vi "Calculate execution time for scans.vi"(8 "error in (no error)":errorcluster, 11 "Command string IN":string) -> (0 "error out":errorcluster, 3 "Execution time":dbl)   [LabVIEW 2012]
doc: "SciScan 1.2 160622"
uses:
  INI/settingsIO/Settings IO_Commands.ctl
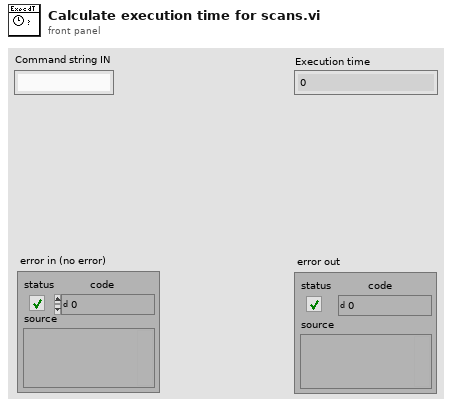
[diagram p1: front panel]
types:
  T1 = typedef "Setting File Types.ctl" = enum16{"2D.Frame.Scan.Settings", "2D.Line.Scan.Settings", "Z.Stack.Settings", "HW Settings", "Configuration Settings", "Unknown Settings", "Fast.Z.Settings"}
  T2 = typedef "Settings IO_Commands.ctl" = enum16{"Write HW Settings", "Write Config Settings", "Read HW Settings", "Read Config Settings", "Write Line-Scan Settings", "Write Frame-Scan Settings", "Write Z-Stack Settings", "Read Line-Scan Settings", "Read Frame-Scan Settings", "Read Z-Stack Settings", "Read Fast-Z Settings", "Write Fast-Z Settings"}
  T3 = typedef "GFG Variable for IO.ctl" = cluster{"Variable Name":string, "Value (Variant)":variant, "data type":string}
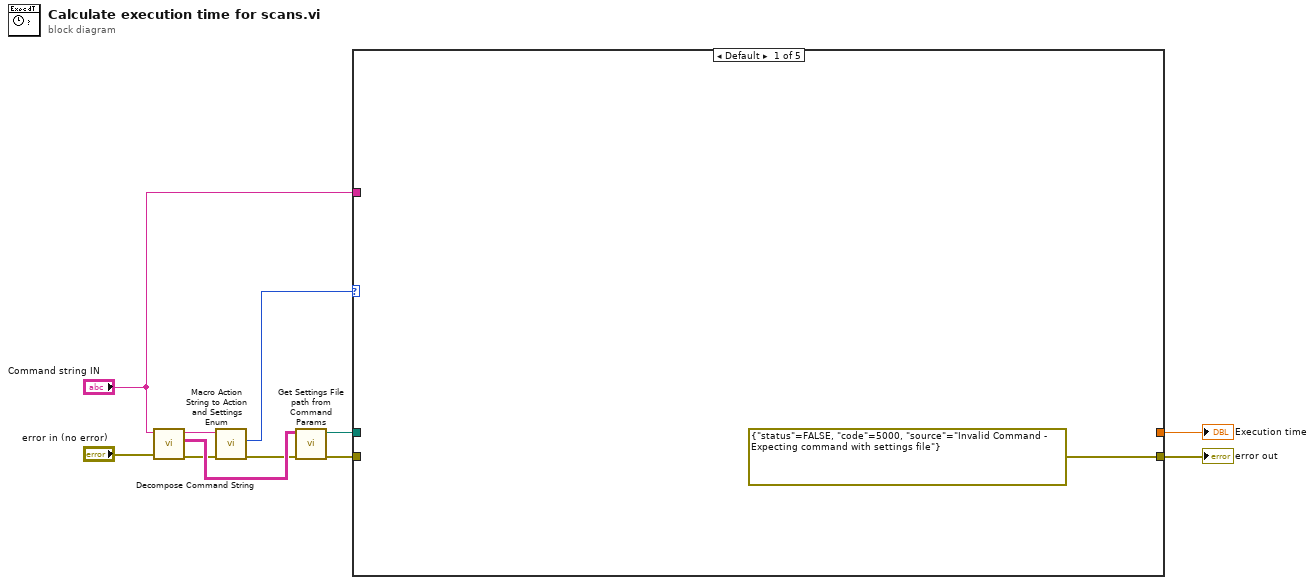
[diagram p0: block diagram]
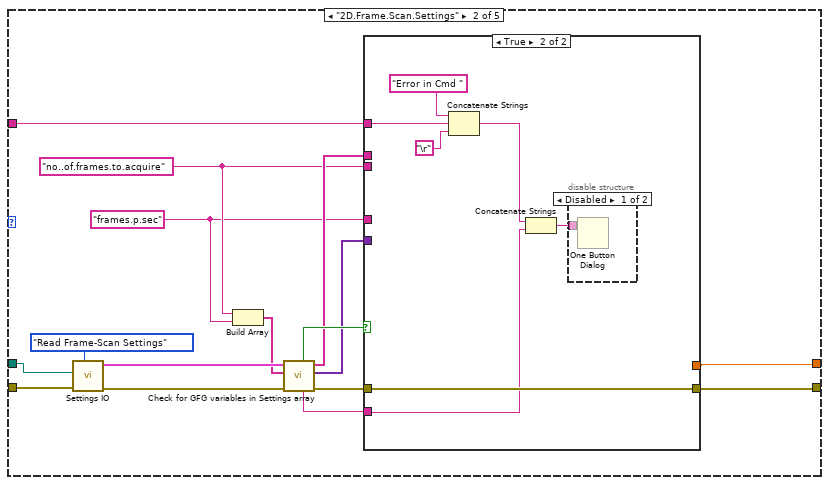
[diagram p2: hidden frame]
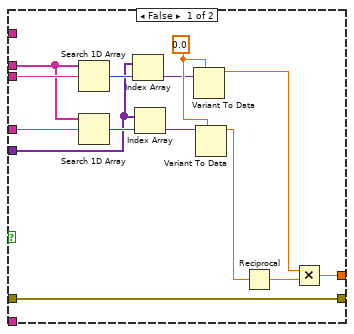
[diagram p3: hidden frame]
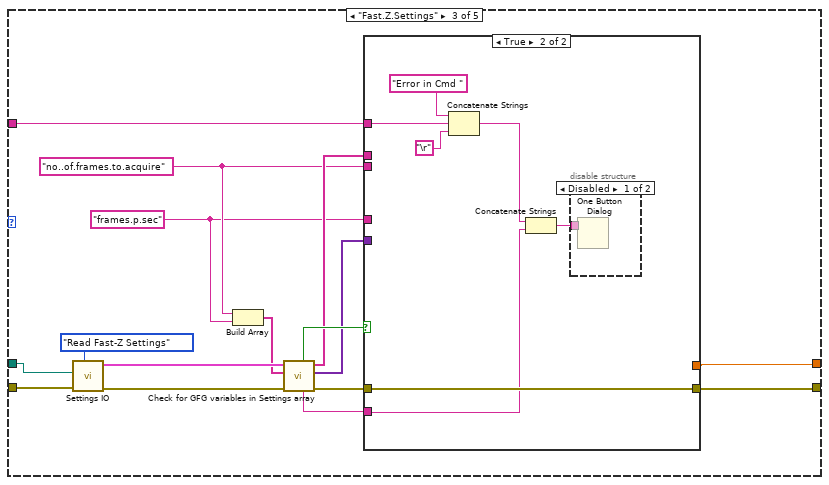
[diagram p5: hidden frame]
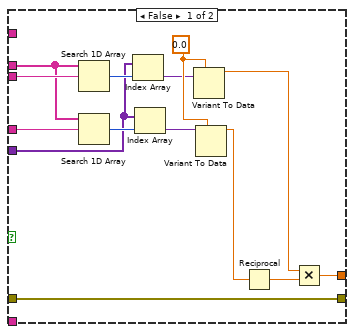
[diagram p6: hidden frame]
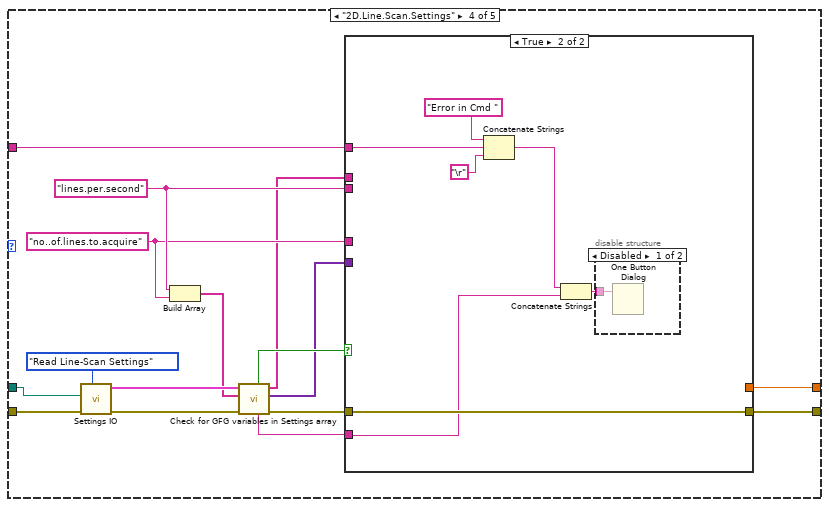
[diagram p8: hidden frame]
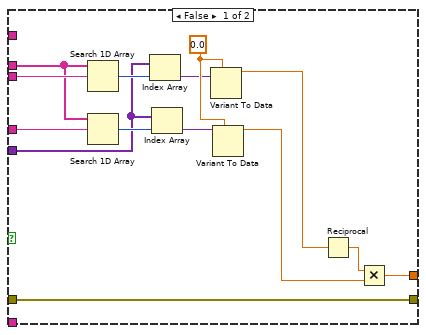
[diagram p9: hidden frame]
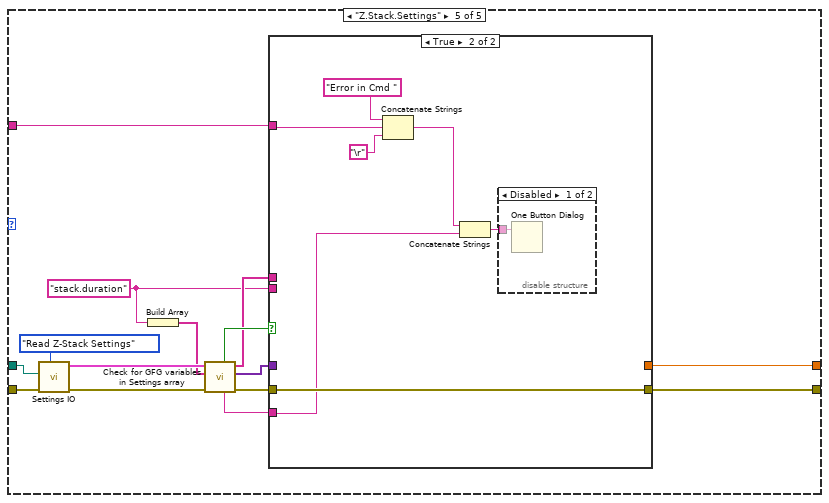
[diagram p11: hidden frame]
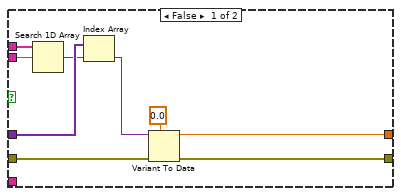
[diagram p12: hidden frame]
diagram:
  n1 = call "Decompose Command String.vi"("Error In"="error in (no error)", "Command IN"="Command string IN") -> ("Error Out"=w10:errorcluster, "Parameter Table"=w11:string[][], "Action"=w9:string)  [unwired: 6 in, 1 out]
  n2 = call "Macro Action String to Action and Settings Enum.vi"("error in (no error)"=w10, "Action String IN"=w9) -> ("error out"=w8:errorcluster, "Setting File Type OUT"=w7:T1)  [unwired: 6 in, 2 out]
  n3 = call "Get Settings File path from Command Params.vi"("error in (no error)"=w8, "Params Array IN"=w11) -> ("error out"=w5:errorcluster, "Settings Path OUT"=w6:path)  [unwired: 8 in]
  n4 = case shown="Default" w7 {
    tunnel: w6 -> [_ w23 w61 w102 w139]
    tunnel: w5 -> [_ w24 w62 w103 w140]
    tunnel: [errorcluster {"status"=FALSE, "code"=5000, "source"="Invalid Command - Expecting command with settings file"} ("error constant") w22 w60 w95 w133] -> w2
    tunnel: [_ w14 w52 w94 w132] -> w4
    tunnel: "Command string IN" -> [_ w13 w51 w89 w127]
    frame Default {
    }
    frame "2D.Frame.Scan.Settings" {
      w17 = "no..of.frames.to.acquire" ("Command string IN 2")
      w16 = "frames.p.sec" ("Command string IN 2")
      n5 = call "Settings IO.vi"("SettingsFileIO_Commands"=Settings_IO_Commands."Read Frame-Scan Settings", "Error In"=w24, "File Path (for scan specific settings)"=w23) -> ("Error Out"=w26:errorcluster, "Settings Array OUT"=w27:T3[])  [unwired: 6 in, 1 out]
      n6 = Build Array(w17, w16) -> (w25:string[])
      n7 = call "Check for GFG variables in Settings array.vi"("error in (no error)"=w26, "GFG variables to search"=w25, "Settings ArrayIN"=w27) -> ("error out"=w21:errorcluster, "GFG variant values (those found)"=w15:variant[], "GFG variables found"=w18:string[], "Error Message (list of variables not found)"=w19:string, "Any Not Found?"=w20:bool)  [unwired: 3 in, 1 out]
      n8 = case shown="True" w20 {
        tunnel: w19 -> [_ w44]
        tunnel: w21 -> [w42 w49]
        tunnel: [w42 w49] -> w22
        tunnel: [w41 _] -> w14
        tunnel: w17 -> [w35 _]
        tunnel: w16 -> [w34 _]
        tunnel: w18 -> [w33 _]
        tunnel: w15 -> [w32 _]
        tunnel: w13 -> [_ w47]
        frame False {
          w40 = 0.0 ("x*y")
          n9 = Search 1D Array(1D array=w33, element=w35) -> (index of element=w37:i32)  [unwired: 1 in]
          n10 = Search 1D Array(1D array=w33, element=w34) -> (index of element=w36:i32)  [unwired: 1 in]
          n11 = Index Array(array=w32, index=w37) -> (element=w39:variant)
          n12 = Index Array(array=w32, index=w36) -> (element=w38:variant)
          n13 = Variant To Data(type=w40, Variant=w39) -> (data=w31:dbl)  [unwired: 1 in, 1 out]
          n14 = Variant To Data(type=w40, Variant=w38) -> (data=w30:dbl)  [unwired: 1 in, 1 out]
          n15 = Reciprocal(x=w30) -> (1/x=w29:dbl)
          n16 = Multiply(x=w31, y=w29) -> (x*y=w41:dbl)
        }
        frame True {
          n17 = Concatenate Strings("Error in Cmd " ("Error Message (list of variables not found)"), w47, "\r") -> (w45:string)
          n18 = Concatenate Strings(w45, w44) -> (w43:string)
          n19 = disable-structure shown="Disabled" {
            disable-tunnel: w43 -> [w50 _]
            frame Disabled {
              n20 = One Button Dialog(message=w50) -> ()  [unwired: 1 in, 1 out]
            }
            frame Enabled {
            }
          }
        }
      }
    }
    frame "Fast.Z.Settings" {
      w55 = "no..of.frames.to.acquire" ("Command string IN 2")
      w54 = "frames.p.sec" ("Command string IN 2")
      n21 = call "Settings IO.vi"("SettingsFileIO_Commands"=Settings_IO_Commands."Read Fast-Z Settings", "Error In"=w62, "File Path (for scan specific settings)"=w61) -> ("Error Out"=w64:errorcluster, "Settings Array OUT"=w65:T3[])  [unwired: 6 in, 1 out]
      n22 = Build Array(w55, w54) -> (w63:string[])
      n23 = call "Check for GFG variables in Settings array.vi"("error in (no error)"=w64, "GFG variables to search"=w63, "Settings ArrayIN"=w65) -> ("error out"=w59:errorcluster, "GFG variant values (those found)"=w53:variant[], "GFG variables found"=w56:string[], "Error Message (list of variables not found)"=w57:string, "Any Not Found?"=w58:bool)  [unwired: 3 in, 1 out]
      n24 = case shown="True" w58 {
        tunnel: w57 -> [_ w82]
        tunnel: w59 -> [w80 w87]
        tunnel: [w80 w87] -> w60
        tunnel: [w79 _] -> w52
        tunnel: w55 -> [w73 _]
        tunnel: w54 -> [w72 _]
        tunnel: w56 -> [w71 _]
        tunnel: w53 -> [w70 _]
        tunnel: w51 -> [_ w85]
        frame False {
          w78 = 0.0 ("x*y")
          n25 = Search 1D Array(1D array=w71, element=w73) -> (index of element=w75:i32)  [unwired: 1 in]
          n26 = Search 1D Array(1D array=w71, element=w72) -> (index of element=w74:i32)  [unwired: 1 in]
          n27 = Index Array(array=w70, index=w75) -> (element=w77:variant)
          n28 = Index Array(array=w70, index=w74) -> (element=w76:variant)
          n29 = Variant To Data(type=w78, Variant=w77) -> (data=w69:dbl)  [unwired: 1 in, 1 out]
          n30 = Variant To Data(type=w78, Variant=w76) -> (data=w68:dbl)  [unwired: 1 in, 1 out]
          n31 = Reciprocal(x=w68) -> (1/x=w67:dbl)
          n32 = Multiply(x=w69, y=w67) -> (x*y=w79:dbl)
        }
        frame True {
          n33 = Concatenate Strings("Error in Cmd " ("Error Message (list of variables not found)"), w85, "\r") -> (w83:string)
          n34 = Concatenate Strings(w83, w82) -> (w81:string)
          n35 = disable-structure shown="Disabled" {
            disable-tunnel: w81 -> [w88 _]
            frame Disabled {
              n36 = One Button Dialog(message=w88) -> ()  [unwired: 1 in, 1 out]
            }
            frame Enabled {
            }
          }
        }
      }
    }
    frame "2D.Line.Scan.Settings" {
      w92 = "no..of.lines.to.acquire" ("Variable Name in")
      w93 = "lines.per.second" ("Variable Name in")
      n37 = call "Settings IO.vi"("SettingsFileIO_Commands"=Settings_IO_Commands."Read Line-Scan Settings", "Error In"=w103, "File Path (for scan specific settings)"=w102) -> ("Error Out"=w98:errorcluster, "Settings Array OUT"=w101:T3[])  [unwired: 6 in, 1 out]
      n38 = Build Array(w93, w92) -> (w96:string[])
      n39 = call "Check for GFG variables in Settings array.vi"("error in (no error)"=w98, "GFG variables to search"=w96, "Settings ArrayIN"=w101) -> ("error out"=w97:errorcluster, "GFG variant values (those found)"=w90:variant[], "GFG variables found"=w91:string[], "Error Message (list of variables not found)"=w99:string, "Any Not Found?"=w100:bool)  [unwired: 3 in, 1 out]
      n40 = case shown="True" w100 {
        tunnel: w99 -> [_ w120]
        tunnel: w97 -> [w118 w125]
        tunnel: [w118 w125] -> w95
        tunnel: [w117 _] -> w94
        tunnel: w93 -> [w111 _]
        tunnel: w92 -> [w110 _]
        tunnel: w91 -> [w109 _]
        tunnel: w90 -> [w108 _]
        tunnel: w89 -> [_ w119]
        frame False {
          w116 = 0.0 ("x*y")
          n41 = Search 1D Array(1D array=w109, element=w111) -> (index of element=w113:i32)  [unwired: 1 in]
          n42 = Search 1D Array(1D array=w109, element=w110) -> (index of element=w112:i32)  [unwired: 1 in]
          n43 = Index Array(array=w108, index=w113) -> (element=w115:variant)
          n44 = Index Array(array=w108, index=w112) -> (element=w114:variant)
          n45 = Variant To Data(type=w116, Variant=w115) -> (data=w106:dbl)  [unwired: 1 in, 1 out]
          n46 = Variant To Data(type=w116, Variant=w114) -> (data=w107:dbl)  [unwired: 1 in, 1 out]
          n47 = Reciprocal(x=w106) -> (1/x=w105:dbl)
          n48 = Multiply(x=w105, y=w107) -> (x*y=w117:dbl)
        }
        frame True {
          n49 = Concatenate Strings("Error in Cmd " ("Error Message (list of variables not found)"), w119, "\r") -> (w122:string)
          n50 = Concatenate Strings(w122, w120) -> (w121:string)
          n51 = disable-structure shown="Disabled" {
            disable-tunnel: w121 -> [w126 _]
            frame Disabled {
              n52 = One Button Dialog(message=w126) -> ()  [unwired: 1 in, 1 out]
            }
            frame Enabled {
            }
          }
        }
      }
    }
    frame "Z.Stack.Settings" {
      w128 = "stack.duration" ("Command string IN 2")
      n53 = call "Settings IO.vi"("SettingsFileIO_Commands"=Settings_IO_Commands."Read Z-Stack Settings", "Error In"=w140, "File Path (for scan specific settings)"=w139) -> ("Error Out"=w137:errorcluster, "Settings Array OUT"=w138:T3[])  [unwired: 6 in, 1 out]
      n54 = Build Array(w128) -> (w131:string[])
      n55 = call "Check for GFG variables in Settings array.vi"("error in (no error)"=w137, "GFG variables to search"=w131, "Settings ArrayIN"=w138) -> ("error out"=w134:errorcluster, "GFG variant values (those found)"=w130:variant[], "GFG variables found"=w129:string[], "Error Message (list of variables not found)"=w135:string, "Any Not Found?"=w136:bool)  [unwired: 3 in, 1 out]
      n56 = case shown="True" w136 {
        tunnel: w135 -> [_ w151]
        tunnel: w134 -> [w149 w157]
        tunnel: [w142 w157] -> w133
        tunnel: [w143 _] -> w132
        tunnel: w130 -> [w146 _]
        tunnel: w129 -> [w148 _]
        tunnel: w128 -> [w147 _]
        tunnel: w127 -> [_ w152]
        frame False {
          n57 = Search 1D Array(1D array=w148, element=w147) -> (index of element=w145:i32)  [unwired: 1 in]
          n58 = Index Array(array=w146, index=w145) -> (element=w144:variant)
          n59 = Variant To Data(error in=w149, type=0.0 ("x*y"), Variant=w144) -> (data=w143:dbl, error out=w142:errorcluster)
        }
        frame True {
          n60 = Concatenate Strings("Error in Cmd " ("Error Message (list of variables not found)"), w152, "\r") -> (w154:string)
          n61 = Concatenate Strings(w154, w151) -> (w153:string)
          n62 = disable-structure shown="Disabled" {
            disable-tunnel: w153 -> [w158 _]
            frame Disabled {
              n63 = One Button Dialog(message=w158) -> ()  [unwired: 1 in, 1 out]
            }
            frame Enabled {
            }
          }
        }
      }
    }
  }
  "error out" <- w2
  "Execution time" <- w4
